vi "Log Prompt Async.vi"(7 "VolatusAPI":refnum<class "VolatusAPI.lvclass">, 11 "LoggingControl in":refnum<class "LoggingControl.lvclass">) -> ()   [LabVIEW 2020, in "VolatusGUIElements.lvlib" / "LoggingControl.lvclass"]
uses:
  LoggingControl.lvclass
  Volatus/VolatusAPI/VolatusAPI.lvclass
  lv-cdm/CDM-Config/ISO8601 Config.ctl
  lv-cdm/CDM-Config/Format.ctl
  lv-cdm/CDM-Config/Precision.ctl
  lv-cdm/CDM-Config/Timezone.ctl
  messages/StartLog/Data.ctl
  Prompt Result.ctl
  Prompt Action.ctl
  LoggingControl.lvclass/LoggingControl.ctl
  messages/StartLog/Class/Msg.lvclass/Msg.ctl
  Volatus/VolatusAPI/VolatusAPI.lvclass/VolatusAPI.ctl
  messages/StartLog/Class/Msg.lvclass
  C:/dev/lv20CE/relink/lv-protoc/LV-Proto/Message/Message.lvclass
  lv-cdm/CDM-Config/ISO-8601 Format Strings.vi
  lv-vecto/Vecto/TCPMessageService/Send Message.vi
  <vilib>/Utility/error.llb/Error Cluster From Error Code.vi
  lv-protoc/LV-Proto/Message/Message.lvclass
  lv-cdm/CDM-Config/CDM-Config.lvlib
  messages/StartLog/StartLog.lvlib
  C:/dev/lv20CE/relink/lv-volatus/messages/StartLog/Class/Msg.lvclass
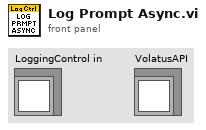
[diagram p1: front panel]
types:
  T1 = typedef "VolatusGUIElements.lvlib/LoggingControl.lvclass/Prompt Action.ctl" = enum16{"Cancelled", "Started"}
  T2 = typedef "VolatusGUIElements.lvlib/LoggingControl.lvclass/Prompt Result.ctl" = cluster{"Action":T1, "Series":string, "Timestamp":string}
  T3 = typedef "StartLog.lvlib/Data.ctl" = cluster{"series":string, "timestamp":string, "started_by":string}
  T4 = typedef "CDM-Config.lvlib/ISO8601 Config.ctl" = cluster{"Format":T5, "Precision":T6, "Timezone":T7}
  T5 = typedef "CDM-Config.lvlib/Format.ctl" = enum16{"Extended", "Basic"}
  T6 = typedef "CDM-Config.lvlib/Precision.ctl" = enum16{"Millisecond", "Second", "Minute", "Hour", "Day"}
  T7 = typedef "CDM-Config.lvlib/Timezone.ctl" = enum16{"UTC", "Local"}
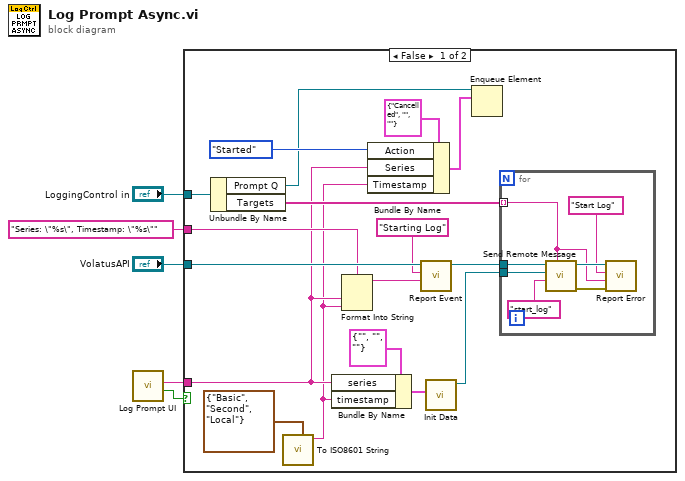
[diagram p0: block diagram]
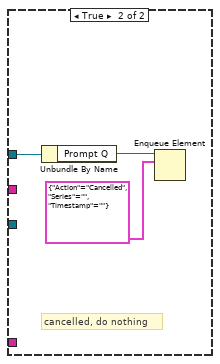
[diagram p2: hidden frame]
diagram:
  n1 = call "Log Prompt UI.vi"() -> ("Cancelled"=w5:bool, "Series"=w4:string)  [unwired: 10 in]
  n2 = case shown="False" w5 {
    tunnel: w4 -> [w7 _]
    tunnel: "LoggingControl in" -> [w19 w32]
    tunnel: "VolatusAPI" -> [w18 _]
    tunnel: "Series: \"%s\", Timestamp: \"%s\"" -> [w8 _]
    frame False {
      n3 = Unbundle By Name(w19) -> ("Prompt Q"=w12:refnum<queue>, "Targets"=w17:string[])
      n4 = call "To ISO8601 String.vi"("Format Config"=T4 {"Format"=enum."Basic", "Precision"=enum."Second", "Timezone"=enum."Local"}) -> ("ISO 8601"=w6:string)  [unwired: 10 in]
      n5 = Bundle By Name(cluster=T3 {"series"="", "timestamp"="", "started_by"=""} ("Data"), "series"=w7, "timestamp"=w6) -> (w20:T3)
      n6 = Format Into String(format string=w8, w7, w6) -> (resulting string=w9:string)  [unwired: 2 in, 1 out]
      n7 = Bundle By Name(cluster=T2 {"Action"=enum."Cancelled", "Series"="", "Timestamp"=""} ("Prompt Result"), "Action"=Prompt_Action."Started", "Series"=w7, "Timestamp"=w6) -> (w15:T2)
      n8 = call "Report Event.vi"("Message"=w9, "Context"="Starting Log", "VolatusAPI in"=w18) -> ("VolatusAPI out"=w11:refnum<class "VolatusAPI.lvclass">)  [unwired: 7 in, 1 out]
      n9 = call "Init Data.vi"("Data"=w20) -> ("Msg out"=w16:refnum<class "Msg.lvclass">)  [unwired: 10 in]
      n10 = Enqueue Element(queue=w12, element=w15) -> ()  [unwired: 2 in, 3 out]
      n11 = for {
        tunnel: w11 -> [w29]
        tunnel: w17 -> [w24] mode=indexing
        tunnel: w16 -> [w28]
        n12 = call "Send Remote Message.vi"("Target Name"=w24, "Message Type"="start_log", "Message"=w28, "VolatusAPI in"=w29) -> ("error out"=w23:errorcluster, "VolatusAPI out"=w26:refnum<class "VolatusAPI.lvclass">)  [unwired: 6 in]
        n13 = call "Report Error.vi"("error in (no error)"=w23, "Message"=w24, "Context"="Start Log", "VolatusAPI in"=w26) -> ()  [unwired: 6 in, 2 out]
      }
    }
    frame True {
      # "cancelled, do nothing"
      n14 = Unbundle By Name(w32) -> ("Prompt Q"=w31:refnum<queue>)
      n15 = Enqueue Element(queue=w31, element=T2 {"Action"=enum."Cancelled", "Series"="", "Timestamp"=""}) -> ()  [unwired: 2 in, 3 out]
    }
  }
